vi "generate_plot_output.vi"(8 "error in (no error)":errorcluster, 11 "Plots in":refnum<class "Plots.lvclass">) -> (0 "error out":errorcluster, 2 "plot array out":cluster{cluster{"X":dbl, "Y":dbl}[]}[](array[cluster]), 3 "Plots out":refnum<class "Plots.lvclass">)   [LabVIEW 2017, in "Plots.lvclass"]
doc: "uses the \"plot data\" (xdata,ydata,flag) from the PlotObject and generates an ouput that can be wired directly into the plot indicator (array for plot unflagged data, array for flagged data, array for fit data)"
uses:
  Plots.lvclass
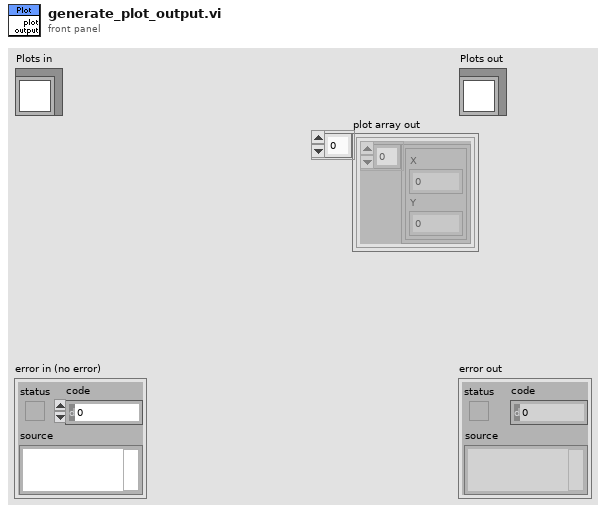
[diagram p1: front panel]
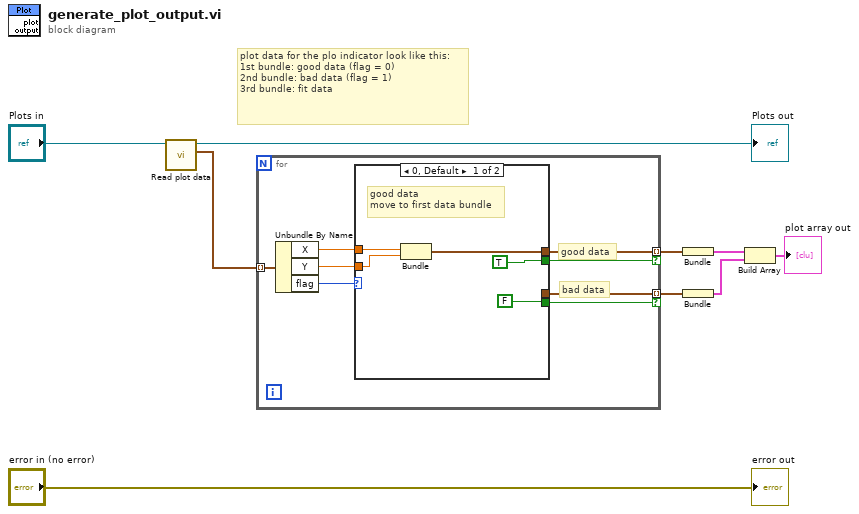
[diagram p0: block diagram]
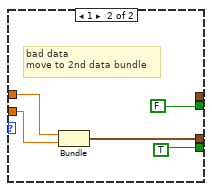
[diagram p2: hidden frame]
diagram:
  # "plot data for the plo indicator look like this:\n1st bundle: good data (flag = 0)\n2nd bundle: bad data (flag = 1)\n3rd bundle: fit data"
  n1 = call-dynamic "Read plot data.vi"("Plots in"="Plots in") -> ("plot data"=w6:cluster{"X":dbl, "Y":dbl, "flag":u8}[], "Plots out"=→"Plots out":refnum<class "Plots.lvclass">)  [unwired: 8 in, 1 out]
  n2 = for {
    tunnel: w6 -> [w17] mode=indexing
    tunnel: [w13] -> w5 mode=indexing if=w12
    tunnel: [w11] -> w4 mode=indexing if=w10
    # "bad data"
    # "good data"
    n3 = Unbundle By Name(w17) -> ("X"=w15:dbl, "Y"=w14:dbl, "flag"=w16:u8)
    n4 = case shown="0, Default" w16 {
      tunnel: w15 -> [w22 w27]
      tunnel: w14 -> [w21 w26]
      tunnel: [w20 _] -> w13
      tunnel: [TRUE FALSE] -> w12
      tunnel: [_ w25] -> w11
      tunnel: [FALSE TRUE] -> w10
      frame 0, Default {
        # "good data\nmove to first data bundle"
        n5 = Bundle("X"=w22, "Y"=w21) -> (w20:cluster{"X":dbl, "Y":dbl})  [unwired: 1 in]
      }
      frame 1 {
        # "bad data\nmove to 2nd data bundle"
        n6 = Bundle("X"=w27, "Y"=w26) -> (w25:cluster{"X":dbl, "Y":dbl})  [unwired: 1 in]
      }
    }
  }
  n7 = Bundle(w5) -> (w3:cluster{cluster{"X":dbl, "Y":dbl}[]})  [unwired: 1 in]
  n8 = Bundle(w4) -> (w2:cluster{cluster{"X":dbl, "Y":dbl}[]})  [unwired: 1 in]
  n9 = Build Array(w3, w2) -> (→"plot array out":cluster{cluster{"X":dbl, "Y":dbl}[]}[])
  "error out" <- "error in (no error)"
